vi "TerminateProcess.vi"(11 "DebuggingTerminal in":refnum<class "DebuggingTerminal.lvclass">) -> (3 "DebuggingTerminal out":refnum<class "DebuggingTerminal.lvclass">)   [LabVIEW 2013, in "MQTT Base.lvlib" / "DebuggingTerminal.lvclass"]
uses:
  DebuggingTerminal.lvclass
  DebuggingTerminal.lvclass/DebuggingTerminal.ctl
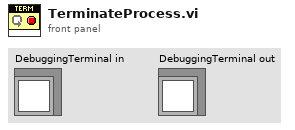
[diagram p1: front panel]
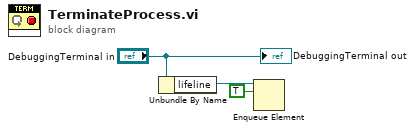
[diagram p0: block diagram]
diagram:
  n1 = Unbundle By Name("DebuggingTerminal in") -> ("lifeline"=w2:refnum<queue>)
  n2 = Enqueue Element(queue=w2, element=TRUE) -> ()  [unwired: 2 in, 3 out]
  "DebuggingTerminal out" <- "DebuggingTerminal in"
